vi "NotaVF.vi"() -> ()   [LabVIEW 2018]
uses:
  <vilib>/Analysis/baseanly.llb/Mean (DBL).vi
  <vilib>/Analysis/NI_AALBase.lvlib
panel:
  out "Nota de VC \n   inválida":bool
  out "Nota de VE \n   inválida":bool
  out "<4?":bool
  out "Nota de VF\n necessária":dbl=nan
  in  "Nota da VC":dbl=nan format="%0.2f"
  out "Média de VE":dbl=nan format="%0.2f"
  in  "Notas de VE":dbl[](array[numeric]) format="%0.2f"
  # "Insira suas notas abaixo"
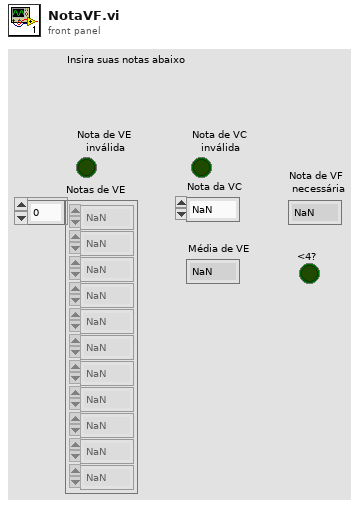
[diagram p1: front panel]
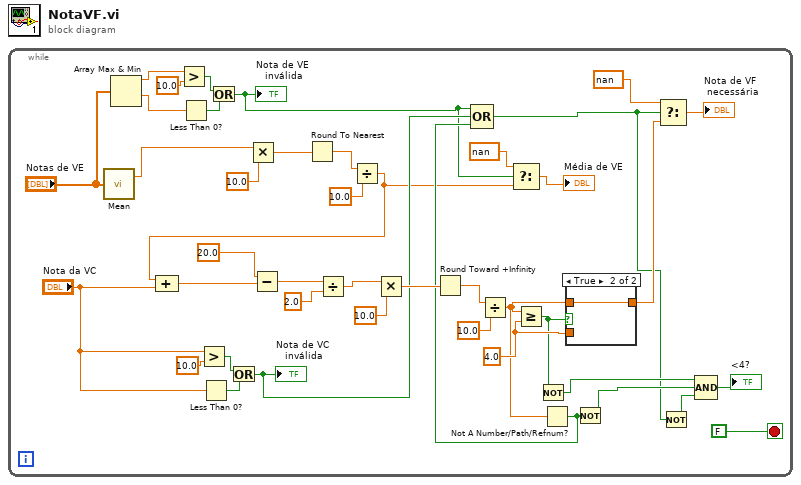
[diagram p0: block diagram]
diagram:
  n1 = while {
    stop <- FALSE stop-if-true
    w32 = 4.0 ("x")
    n2 = call-poly <vilib>:"Mean.vi"("X"="Notas de VE") -> ("mean"=w26:dbl)  [unwired: 1 out]
    n3 = Array Max & Min(array="Notas de VE") -> (max value=w24:dbl, min value=w22:dbl)  [unwired: 2 out]
    n4 = Greater?(x=w24, y=10.0 ("x")) -> (0:w20:bool)
    n5 = Less Than 0?(x=w22) -> (x < 0?=w21:bool)
    n6 = Greater?(x="Nota da VC", y=10.0 ("x")) -> (0:w17:bool)
    n7 = Less Than 0?(x="Nota da VC") -> (x < 0?=w18:bool)
    n8 = Or(x=w20, y=w21) -> (x .or. y?=w3:bool)
    "Nota de VE \n   inválida" <- w3
    n9 = Or(x=w17, y=w18) -> (x .or. y?=w15:bool)
    "Nota de VC \n   inválida" <- w15
    n10 = Multiply(x=w26, y=10.0 ("x")) -> (x*y=w29:dbl)
    n11 = Round To Nearest(number=w29) -> (nearest integer value=w30:dbl)
    n12 = Divide(x=w30, y=10.0 ("x")) -> (x/y=w4:dbl)
    n13 = Compound Arithmetic op=ADD(w4, "Nota da VC") -> (w41:dbl)
    n14 = Subtract(x=20.0, y=w41) -> (x-y=w39:dbl)
    n15 = Divide(x=w39, y=2.0 ("x")) -> (x/y=w34:dbl)
    n16 = Multiply(x=w34, y=10.0 ("x")) -> (x*y=w37:dbl)
    n17 = Round Toward +Infinity(x=w37) -> (ceil(x): smallest int >= x=w38:dbl)
    n18 = Divide(x=w38, y=10.0 ("x")) -> (x/y=w11:dbl)
    n19 = Select(t=nan ("number/path/refnum"), s=w3, f=w4) -> (s? t:f=→"Média de VE":dbl)
    n20 = Greater Or Equal?(x=w11, y=w32) -> (x >= y?=w31:bool)
    n21 = Not(x=w31) -> (.not. x?=w9:bool)
    n22 = Not A Number/Path/Refnum?(number/path/refnum=w11) -> (NaN/Path/Refnum?=w7:bool)
    n23 = Compound Arithmetic op=OR(w3, w15, w7) -> (w6:bool)
    n24 = case shown="True" w31 {
      tunnel: w11 -> [_ w44]
      tunnel: [w43 w44] -> w14
      tunnel: w32 -> [w43 _]
      frame False {
      }
      frame True {
      }
    }
    n25 = Not(x=w7) -> (.not. x?=w10:bool)
    n26 = Select(t=nan ("number/path/refnum"), s=w6, f=w14) -> (s? t:f=→"Nota de VF\n necessária":dbl)
    n27 = Not(x=w6) -> (.not. x?=w5:bool)
    n28 = Compound Arithmetic op=AND(w9, w10, w5) -> (→"<4?":bool)
  }
